vi "Main.vi"() -> ()   [LabVIEW 2020]
uses:
  Libraries/Raster/Screen Dimensions.ctl
  Libraries/3D/Camera.ctl
  <vilib>/Utility/miscctls.llb/LVBoundsTypeDef.ctl
  Libraries/3D/Triangle 3D.ctl
  Libraries/3D/Vector 3D.ctl
  Libraries/3D/3D.lvlib
  Libraries/Raster/Raster.lvlib
panel:
  in  "Update":bool=TRUE
  in  "z Rotation":sgl(slide)=2.6797385 scale=-90.0..90.0
  in  "y Rotation":sgl(slide)=2.6797385 scale=-90.0..90.0
  in  "x Rotation":sgl(slide)=2.6797385 scale=-90.0..90.0
  out "Frame Rate [FPS]":dbl format="%.1p"
  in  "Draw Lines":bool
  in  "Fill Colour":u32(colorbox)=12517256
  in  "Line Colour":u32(colorbox)=4375295
  in  "z Translation":sgl(slide)=2.6797385 scale=0.0..10.0
  out "Delta Time [s]":dbl format="%.3p"
  in  "Camera":T1={"Field Of View"=90.0, "Near Plane"=0.1, "Far Plane"=1000.0}
  in  "Screen Dimensions":T2={"Width"=640, "Height"=480}
  out "Screen":picture
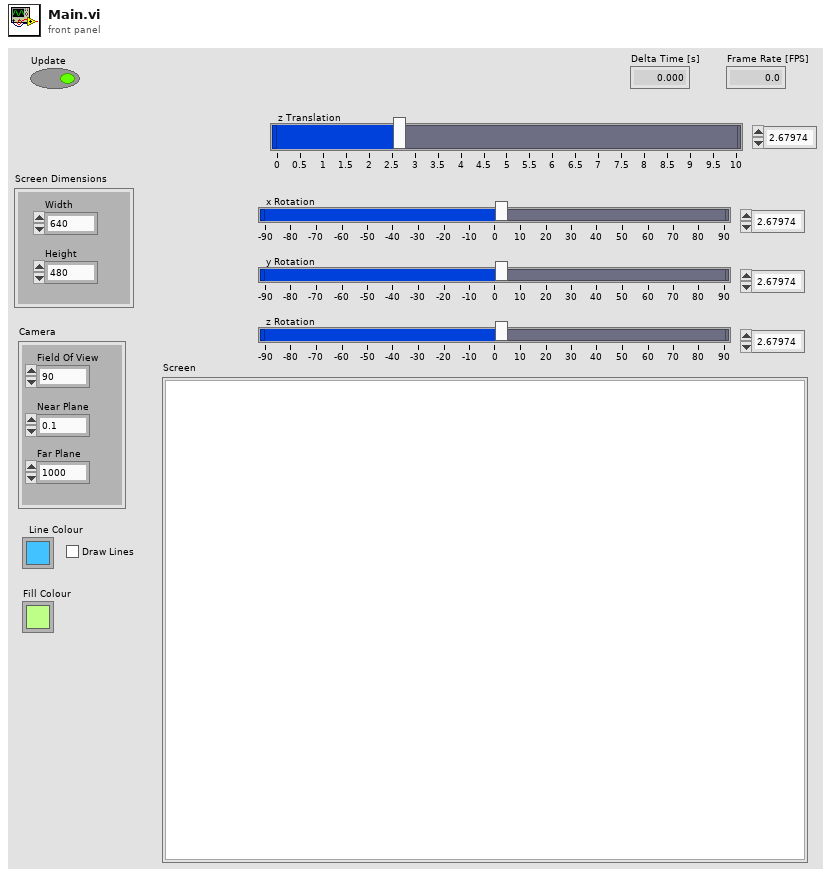
[diagram p1: front panel]
types:
  T1 = typedef "3D.lvlib/Camera.ctl" = cluster{"Field Of View":sgl, "Near Plane":sgl, "Far Plane":sgl}
  T2 = typedef "Raster.lvlib/Screen Dimensions.ctl" = cluster{"Width":u32, "Height":u32}
  T3 = typedef "LVBoundsTypeDef.ctl" = cluster{"Width":u32, "Height":u32}
  T4 = typedef "3D.lvlib/Mesh.ctl" = cluster{"Triangles":T5[]}
  T5 = typedef "3D.lvlib/Triangle 3D.ctl" = cluster{"Point 1":T6, "Point 2":T6, "Point 3":T6, "Fill Colour":u32}
  T6 = typedef "3D.lvlib/Vector 3D.ctl" = cluster{"x":sgl, "y":sgl, "z":sgl}
  T7 = typedef "3D.lvlib/Triangle 2D.ctl" = cluster{"Point 1":T8, "Point 2":T8, "Point 3":T8, "Fill Colour":u32}
  T8 = typedef "3D.lvlib/Point 2D.ctl" = cluster{"x":sgl, "y":sgl}
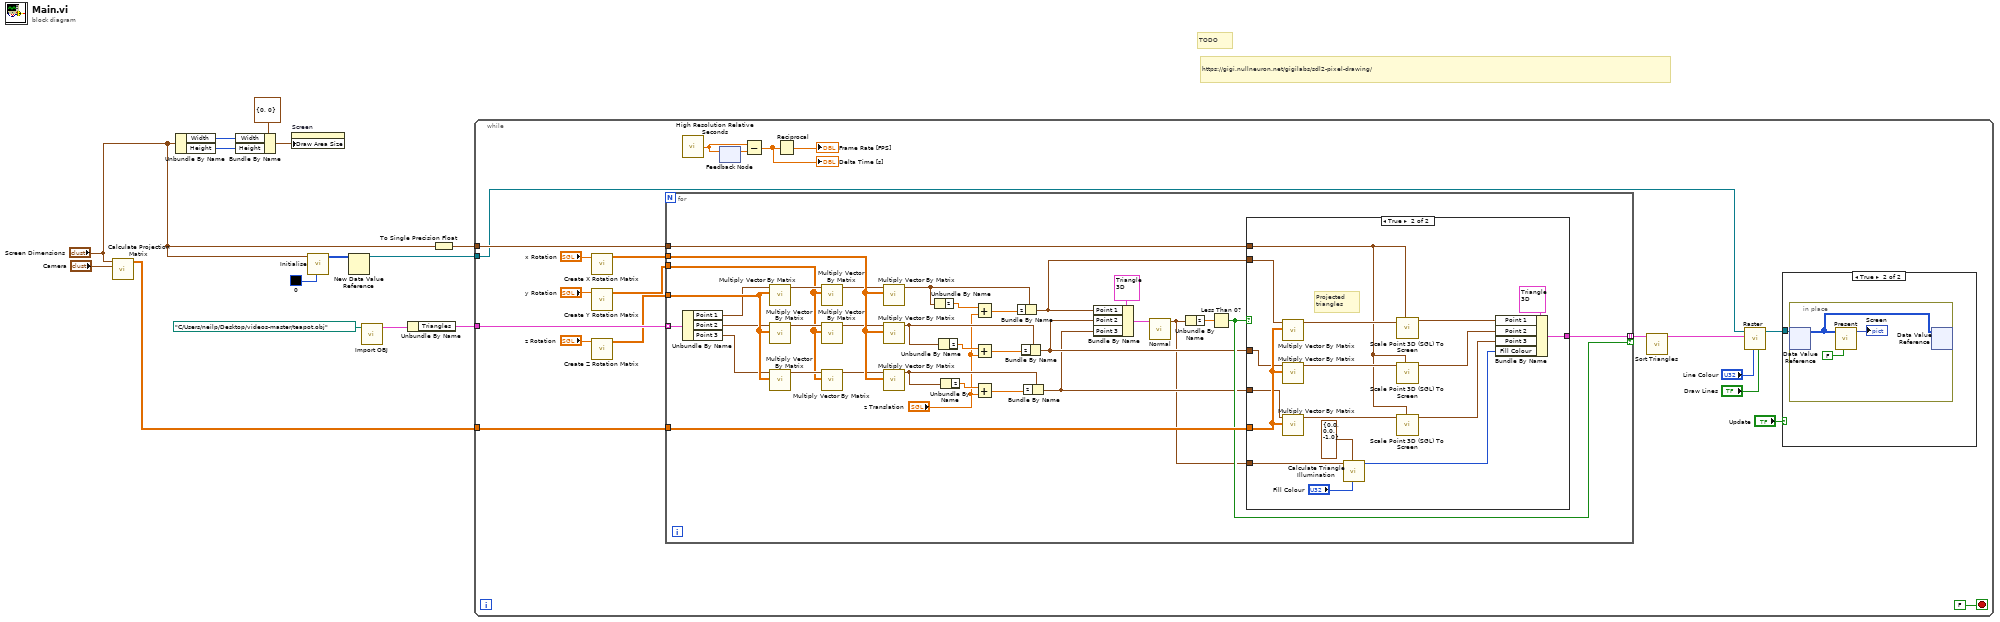
[diagram p0: block diagram]
diagram:
  # "TODO"
  # "https://gigi.nullneuron.net/gigilabs/sdl2-pixel-drawing/"
  n1 = call "Calculate Projection Matrix.vi"("Camera"="Camera", "Screen Dimensions"="Screen Dimensions") -> ("Projection Matrix"=w9:sgl[][])  [unwired: 9 in]
  n2 = Unbundle By Name("Screen Dimensions") -> ("Width"=w12:u32, "Height"=w11:u32)
  n3 = Bundle By Name(cluster=T3 {"Width"=0, "Height"=0} ("Draw Area Size"), "Width"=w12, "Height"=w11) -> (w13:T3)
  n4 = property on="Screen" class="Pict"("Draw Area Size"=w13) -> ()  [unwired: 2 in, 2 out]
  n5 = call "Initialise.vi"("Fill Colour"=u32 0, "Screen Dimensions"="Screen Dimensions") -> ("Pixel Data out"=w5:u32[][])  [unwired: 9 in]
  n6 = New Data Value Reference(data value=w5) -> (data value reference=w4:refnum<data-value>)  [unwired: 1 in, 1 out]
  n7 = call "Import OBJ.vi"("Object"=path "C:/Users/neilp/Desktop/videos-master/teapot.obj") -> ("Object"=w2:T4)  [unwired: 10 in]
  n8 = Unbundle By Name(w2) -> ("Triangles"=w1:T5[])
  n9 = To Single Precision Float(number="Screen Dimensions") -> (single precision float=w6:cluster{"Width":sgl, "Height":sgl})
  n10 = while {
    tunnel: w1 -> [w35]
    tunnel: w9 -> [w34]
    tunnel: w6 -> [w33]
    tunnel: w4 -> [w28]
    stop <- FALSE stop-if-true
    n11 = call "Create X Rotation Matrix.vi"("Theta (°)"="x Rotation") -> ("Rotation X Matrix"=w20:sgl[][])  [unwired: 10 in]
    n12 = call "Create Y Rotation Matrix.vi"("Theta (°)"="y Rotation") -> ("Rotation Y Matrix"=w16:sgl[][])  [unwired: 10 in]
    n13 = call "Create Z Rotation Matrix.vi"("Theta (°)"="z Rotation") -> ("Rotation Z Matrix"=w21:sgl[][])  [unwired: 10 in]
    n14 = for {
      tunnel: w35 -> [w69] mode=indexing
      tunnel: w34 -> [w73]
      tunnel: w33 -> [w72]
      tunnel: w21 -> [w71]
      tunnel: w20 -> [w70]
      tunnel: [w56] -> w29 mode=indexing if=w55
      tunnel: w16 -> [w40]
      n15 = Unbundle By Name(w69) -> ("Point 1"=w54:T6, "Point 2"=w53:T6, "Point 3"=w52:T6)
      n16 = call "Multiply Vector By Matrix.vi"("Matrix in"=w71, "Vector 3D in"=w54) -> ("Vector 3D out"=w46:T6)  [unwired: 9 in]
      n17 = call "Multiply Vector By Matrix.vi"("Matrix in"=w71, "Vector 3D in"=w53) -> ("Vector 3D out"=w44:T6)  [unwired: 9 in]
      n18 = call "Multiply Vector By Matrix.vi"("Matrix in"=w71, "Vector 3D in"=w52) -> ("Vector 3D out"=w42:T6)  [unwired: 9 in]
      n19 = call "Multiply Vector By Matrix.vi"("Matrix in"=w40, "Vector 3D in"=w46) -> ("Vector 3D out"=w45:T6)  [unwired: 9 in]
      n20 = call "Multiply Vector By Matrix.vi"("Matrix in"=w40, "Vector 3D in"=w44) -> ("Vector 3D out"=w43:T6)  [unwired: 9 in]
      n21 = call "Multiply Vector By Matrix.vi"("Matrix in"=w40, "Vector 3D in"=w42) -> ("Vector 3D out"=w41:T6)  [unwired: 9 in]
      n22 = call "Multiply Vector By Matrix.vi"("Matrix in"=w70, "Vector 3D in"=w45) -> ("Vector 3D out"=w66:T6)  [unwired: 9 in]
      n23 = call "Multiply Vector By Matrix.vi"("Matrix in"=w70, "Vector 3D in"=w43) -> ("Vector 3D out"=w61:T6)  [unwired: 9 in]
      n24 = call "Multiply Vector By Matrix.vi"("Matrix in"=w70, "Vector 3D in"=w41) -> ("Vector 3D out"=w60:T6)  [unwired: 9 in]
      n25 = Unbundle By Name(w66) -> ("z"=w68:sgl)
      n26 = Unbundle By Name(w61) -> ("z"=w64:sgl)
      n27 = Unbundle By Name(w60) -> ("z"=w63:sgl)
      n28 = Add(x=w68, y="z Translation") -> (x+y=w67:sgl)
      n29 = Add(x=w64, y="z Translation") -> (x+y=w65:sgl)
      n30 = Add(x=w63, y="z Translation") -> (x+y=w62:sgl)
      n31 = Bundle By Name(cluster=w66, "z"=w67) -> (w51:T6)
      n32 = Bundle By Name(cluster=w61, "z"=w65) -> (w50:T6)
      n33 = Bundle By Name(cluster=w60, "z"=w62) -> (w49:T6)
      n34 = Bundle By Name(cluster=T5 {"Point 1"={"x"=0.0, "y"=0.0, "z"=0.0}, "Point 2"={"x"=0.0, "y"=0.0, "z"=0.0}, "Point 3"={"x"=0.0, "y"=0.0, "z"=0.0}, "Fill Colour"=12517256} ("Triangle"), "Point 1"=w51, "Point 2"=w50, "Point 3"=w49) -> (w48:T5)
      n35 = call "Normal.vi"("Triangle"=w48) -> ("Normal"=w47:T6)  [unwired: 10 in]
      n36 = Unbundle By Name(w47) -> ("z"=w58:sgl)
      n37 = Less Than 0?(x=w58) -> (x < 0?=w55:bool)
      n38 = case shown="True" w55 {
        tunnel: w73 -> [_ w90]
        tunnel: w72 -> [_ w78]
        tunnel: w51 -> [_ w89]
        tunnel: w50 -> [_ w88]
        tunnel: w49 -> [_ w87]
        tunnel: [_ w85] -> w56
        tunnel: w47 -> [_ w77]
        frame False {
        }
        frame True {
          # "Projected triangles"
          n39 = call "Multiply Vector By Matrix.vi"("Matrix in"=w90, "Vector 3D in"=w89) -> ("Vector 3D out"=w79:T6)  [unwired: 9 in]
          n40 = call "Multiply Vector By Matrix.vi"("Matrix in"=w90, "Vector 3D in"=w88) -> ("Vector 3D out"=w81:T6)  [unwired: 9 in]
          n41 = call "Multiply Vector By Matrix.vi"("Matrix in"=w90, "Vector 3D in"=w87) -> ("Vector 3D out"=w80:T6)  [unwired: 9 in]
          n42 = call "Calculate Triangle Illumination.vi"("Fill Colour"="Fill Colour", "Light Direction"=T6 {"x"=0.0, "y"=0.0, "z"=-1.0}, "Triangle Normal"=w77) -> ("Fill Colour Actual"=w75:u32)  [unwired: 8 in]
          n43 = call "Scale Point 3D (SGL) To Screen.vi"("Screen Dimensions"=w78, "Point In"=w79) -> ("Point Out"=w84:T6)  [unwired: 9 in]
          n44 = call "Scale Point 3D (SGL) To Screen.vi"("Screen Dimensions"=w78, "Point In"=w81) -> ("Point Out"=w83:T6)  [unwired: 9 in]
          n45 = call "Scale Point 3D (SGL) To Screen.vi"("Screen Dimensions"=w78, "Point In"=w80) -> ("Point Out"=w82:T6)  [unwired: 9 in]
          n46 = Bundle By Name(cluster=T5 {"Point 1"={"x"=0.0, "y"=0.0, "z"=0.0}, "Point 2"={"x"=0.0, "y"=0.0, "z"=0.0}, "Point 3"={"x"=0.0, "y"=0.0, "z"=0.0}, "Fill Colour"=12517256} ("Triangle"), "Point 1"=w84, "Point 2"=w83, "Point 3"=w82, "Fill Colour"=w75) -> (w85:T5)
        }
      }
    }
    n47 = call <vilib>:"High Resolution Relative Seconds.vi"() -> ("relative seconds"=w31:dbl)
    n48 = feedback-in #1(w31) -> ()
    n49 = feedback #1() -> (w30:dbl)  [unwired: 1 in]
    n50 = Subtract(x=w31, y=w30) -> (x-y=w23:dbl)
    "Delta Time [s]" <- w23
    n51 = Reciprocal(x=w23) -> (1/x=→"Frame Rate [FPS]":dbl)
    n52 = call "Sort Triangles.vi"("Triangles"=w29) -> ("Triangles Sorted"=w27:T7[])  [unwired: 10 in]
    n53 = call "Raster.vi"("Draw Lines"="Draw Lines", "Line Colour"="Line Colour", "Triangles Sorted"=w27, "Pixels"=w28) -> ("Pixels (dup)"=w24:refnum<data-value>)  [unwired: 7 in]
    n54 = case shown="True" "Update" {
      tunnel: w24 -> [_ w36]
      frame False {
      }
      frame True {
        n55 = in-place {
          n56 = in-place-dvr #2(w36) -> (w37:u32[][])  [unwired: 1 out]
          n57 = call "Present.vi"("Reverse Rows (T)"=FALSE, "Pixel Data in"=w37) -> ("2D Picture"=→"Screen":picture)  [unwired: 9 in]
          n58 = in-place-dvr #2(w37) -> ()  [unwired: 2 out]
        }
      }
    }
  }
